vi "Ctor.vi"(8 "error in (no error)":errorcluster, 11 "DB File":path) -> (0 "error out":errorcluster, 3 "SQLite out":refnum<class "SQLite.lvclass">)   [LabVIEW 2020, in "Summer of LabVIEW.lvlib" / "SQLite.lvclass"]
uses:
  SQLite.lvclass
  SQLite.lvclass/SQLite.ctl
  <vilib>/drjdpowell/SQLite Library/SQL Connection/Connection.lvclass
  <vilib>/drjdpowell/SQLite Library/SQLite.lvlib
  <vilib>/drjdpowell/SQLite Library/SQL Connection/Open (path).vi
  <vilib>/drjdpowell/SQLite Library/SQL Connection/Execute SQL (No results).vi
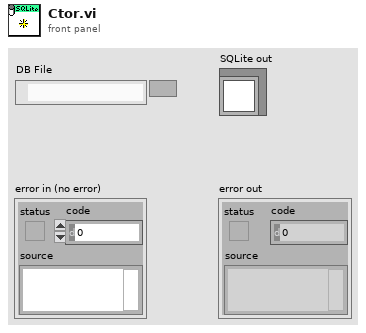
[diagram p1: front panel]
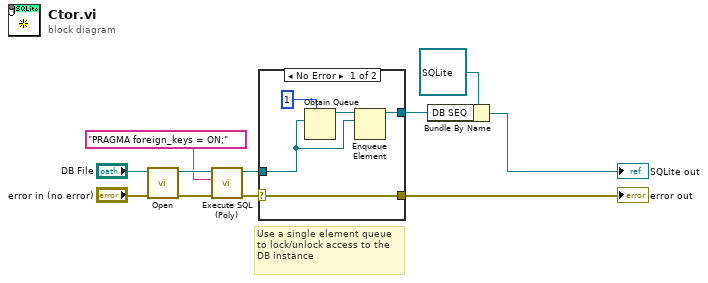
[diagram p0: block diagram]
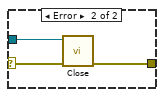
[diagram p2: hidden frame]
diagram:
  # "Use a single element queue to lock/unlock access to the DB instance"
  n1 = call-poly <vilib>:"Open.vi"("error in (no error)"="error in (no error)", "db file"="DB File") -> ("error out"=w4:errorcluster, "SQLite Connection"=w5:refnum<class "Connection.lvclass">)  [unwired: 8 in]
  n2 = call-poly <vilib>:"Execute SQL (Poly).vi"("error in (no error)"=w4, "SQL"="PRAGMA foreign_keys = ON;", "SQLite Connection in"=w5) -> ("error out"=w1:errorcluster, "SQLite Connection"=w2:refnum<class "Connection.lvclass">)  [unwired: 7 in]
  n3 = case shown="No Error" w1 {
    selector: w1 -> [w13 w19]
    tunnel: w2 -> [w12 w18]
    tunnel: [w13 w17] -> w8
    tunnel: [w14 _] -> w6
    frame No Error {
      n4 = Obtain Queue(max queue size (-1, unlimited)=1, element data type=w12) -> (queue out=w15:refnum<queue>)  [unwired: 3 in, 2 out]
      n5 = Enqueue Element(queue=w15, element=w12) -> (queue out=w14:refnum<queue>)  [unwired: 2 in, 2 out]
    }
    frame Error {
      n6 = call-dynamic "Close.vi"("error in (no error)"=w19, "SQLite Connection in"=w18) -> ("error out"=w17:errorcluster)  [unwired: 9 in]
    }
  }
  "error out" <- w8
  n7 = Bundle By Name(cluster=refnum<class "SQLite.lvclass"> refnum ("SQLite in"), "DB SEQ"=w6) -> (→"SQLite out":refnum<class "SQLite.lvclass">)
